vi "SPARK Create.vi"(8 "error in (no error)":errorcluster, 9 "Invert":bool, 10 "Device Number":u8) -> (0 "error out":errorcluster, 3 "MotorControlDeviceRef":T1={"DeviceStatus"={"status"=FALSE, "code"=0, "source"=""}, "Type"=enum."PWM", "PWM"={"PWM Channel"=enum."Invalid", "DeadBand"={"Name"="", "maxPositivePwm"=0, "minPositivePwm"=0, "centerPwm"=0, "maxNegativePwm"=0, "minNegativePwm"=0, "angularRange"=0}}, "CAN"={"Device Number"=0, "SetOutput VI Ref"=variant, "GetOutput VI Ref"=variant, "Enable VI Ref"=variant, "Disable VI Ref"=variant, "Data"=variant}, "Invert"=FALSE, "DIO PWM"={"PWM \"Enable\" Channel"=enum."Invalid", "DIOChannel"=enum."Invalid", "PWM Rate"=0.0}})   [LabVIEW 2023]
doc: "Open the SPARK motor controller.\n\n<b>Device Number</b> is the CAN ID of the controller. Use a value between 1 and 62.\n\n<b>Invert</b> will tell the LabVIEW driver to invert the output of the motor. For a device that is configured as a Follower, this flag will configure the follower to driver opposite of the Leader controller."
uses:
  <vilib>/Rock Robotics/WPI/MotorControl/WPI_MotorControlDeviceRef.ctl
  <vilib>/Rock Robotics/WPI/MotorControl/WPI_MotorControlType.ctl
  <vilib>/Rock Robotics/SystemInterfaces/DIO/FPGA_DIOPWMChannel.ctl
  <vilib>/Rock Robotics/WPI/PWM/WPI_PWMDeadband.ctl
  <vilib>/Rock Robotics/SystemInterfaces/DIO/FPGA_DIOChannel.ctl
  Typedef/Spark MAX Variant Data.ctl
  Typedef/SPARK Model.ctl
  Typedef/SPARK Parameter ID.ctl
  <vilib>/Rock Robotics/SystemInterfaces/NetworkCommunication/NetComm_UsageReport_ResourceType.ctl
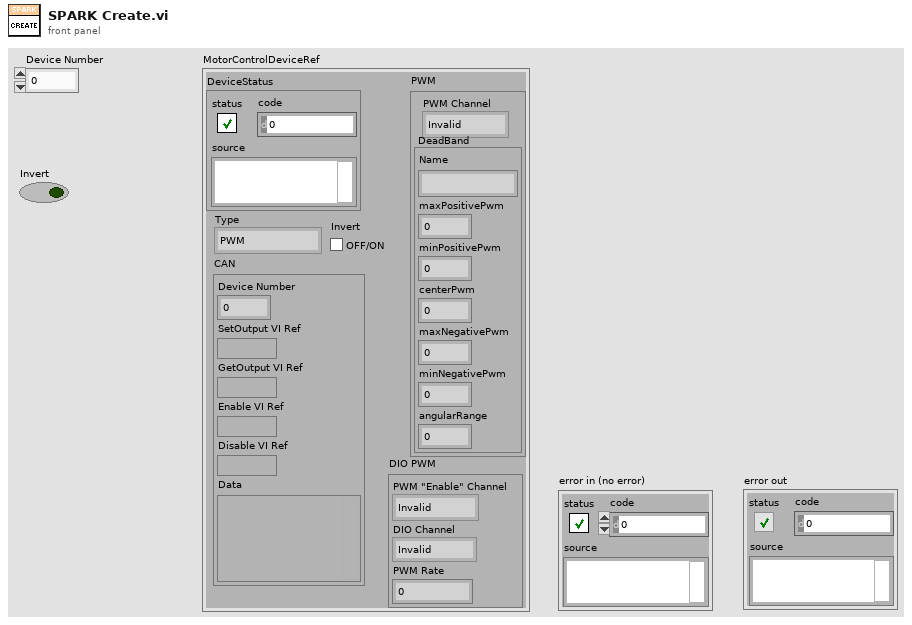
[diagram p1: front panel]
types:
  T1 = typedef "WPI_MotorControlDeviceRef.ctl" = cluster{"DeviceStatus":errorcluster, "Type":T2, "PWM":cluster{"PWM Channel":T3, "DeadBand":T4}, "CAN":cluster{"Device Number":u8, "SetOutput VI Ref":variant, "GetOutput VI Ref":variant, "Enable VI Ref":variant, "Disable VI Ref":variant, "Data":variant}, "Invert":bool, "DIO PWM":cluster{"PWM \"Enable\" Channel":T3, "DIOChannel":T5, "PWM Rate":dbl}}
  T2 = typedef "WPI_MotorControlType.ctl" = enum16{"PWM", "CAN", "DIO PWM"}
  T3 = typedef "FPGA_DIOPWMChannel.ctl" = enum8{"PWM 0", "PWM 1", "PWM 2", "PWM 3", "PWM 4", "PWM 5", "PWM 6", "PWM 7", "PWM 8", "PWM 9", "PWM MXP 0", "PWM MXP 1", "PWM MXP 2", "PWM MXP 3", "PWM MXP 4", "PWM MXP 5", "PWM MXP 6", "PWM MXP 7", "PWM MXP 8", "PWM MXP 9", "Invalid"}
  T4 = typedef "WPI_PWMDeadband.ctl" = cluster{"Name":string, "maxPositivePwm":i32, "minPositivePwm":i32, "centerPwm":i32, "maxNegativePwm":i32, "minNegativePwm":i32, "angularRange":u16}
  T5 = typedef "FPGA_DIOChannel.ctl" = enum8{"DIO 0", "DIO 1", "DIO 2", "DIO 3", "DIO 4", "DIO 5", "DIO 6", "DIO 7", "DIO 8", "DIO 9", "DIO MXP 0", "DIO MXP 1", "DIO MXP 2", "DIO MXP 3", "DIO MXP 4", "DIO MXP 5", "DIO MXP 6", "DIO MXP 7", "DIO MXP 8", "DIO MXP 9", "DIO MXP 10", "DIO MXP 11", "DIO MXP 12", "DIO MXP 13", "DIO MXP 14", "DIO MXP 15", "SPI Port CS1", "SPI Port CS2", "SPI Port CS3", "SPI Port MISO", "SPI Port MOSI", "Invalid"}
  T6 = typedef "SPARK Parameter ID.ctl" = enum16{"kCanID", "kInputMode", "kMotorType", "kCommAdvance", "kSensorType", "kCtrlType", "kIdleMode", "kInputDeadband", "kLegacyFeedbackSensorPID0", "kClosedLoopControlSensor", "kPolePairs", "kCurrentChop", "kCurrentChopCycles", "kP_0", "kI_0", "kD_0", "kF_0", "kIZone_0", "kDFilter_0", "kOutputMin_0", "kOutputMax_0", "kP_1", "kI_1", "kD_1", "kF_1", "kIZone_1", "kDFilter_1", "kOutputMin_1", "kOutputMax_1", "kP_2", "kI_2", "kD_2", "kF_2", "kIZone_2", "kDFilter_2", "kOutputMin_2", "kOutputMax_2", "kP_3", "kI_3", "kD_3", "kF_3", "kIZone_3", "kDFilter_3", "kOutputMin_3", "kOutputMax_3", "kInverted", "kOutputRatio", "kSerialNumberLow", "kSerialNumberMid", "kSerialNumberHigh", "kLimitSwitchFwdPolarity", "kLimitSwitchRevPolarity", "kHardLimitFwdEn", "kHardLimitRevEn", "kSoftLimitFwdEn", "kSoftLimitRevEn", "kRampRate", "kFollowerID", "kFollowerConfig", "kSmartCurrentStallLimit", "kSmartCurrentFreeLimit", "kSmartCurrentConfig", "kSmartCurrentReserved", "kMotorKv", "kMotorR", "kMotorL", "kMotorRsvd1", "kMotorRsvd2", "kMotorRsvd3", "kEncoderCountsPerRev", "kEncoderAverageDepth", "kEncoderSampleDelta", "kEncoderInverted", "kEncoderRsvd1", "kClosedLoopVoltageMode", "kCompensatedNominalVoltage", "kSmartMotionMaxVelocity_0", "kSmartMotionMaxAccel_0", "kSmartMotionMinVelOutput_0", "kSmartMotionAllowedClosedLoopError_0", "kSmartMotionAccelStrategy_0", "kSmartMotionMaxVelocity_1", "kSmartMotionMaxAccel_1", "kSmartMotionMinVelOutput_1", "kSmartMotionAllowedClosedLoopError_1", "kSmartMotionAccelStrategy_1", "kSmartMotionMaxVelocity_2", "kSmartMotionMaxAccel_2", "kSmartMotionMinVelOutput_2", "kSmartMotionAllowedClosedLoopError_2", "kSmartMotionAccelStrategy_2", "kSmartMotionMaxVelocity_3", "kSmartMotionMaxAccel_3", "kSmartMotionMinVelOutput_3", "kSmartMotionAllowedClosedLoopError_3", "kSmartMotionAccelStrategy_3", "kIMaxAccum_0", "kSlot3Placeholder1_0", "kSlot3Placeholder2_0", "kSlot3Placeholder3_0", "kIMaxAccum_1", "kSlot3Placeholder1_1", "kSlot3Placeholder2_1", "kSlot3Placeholder3_1", "kIMaxAccum_2", "kSlot3Placeholder1_2", "kSlot3Placeholder2_2", "kSlot3Placeholder3_2", "kIMaxAccum_3", "kSlot3Placeholder1_3", "kSlot3Placeholder2_3", "kSlot3Placeholder3_3", "kPositionConversionFactor", "kVelocityConversionFactor", "kClosedLoopRampRate", "kSoftLimitFwd", "kSoftLimitRev", "kSoftLimitRsvd0", "kSoftLimitRsvd1", "kAnalogPositionConversion", "kAnalogVelocityConversion", "kAnalogAverageDepth", "kAnalogSensorMode", "kAnalogInverted", "kAnalogSampleDelta", "kAnalogRsvd0", "kAnalogRsvd1", "kDataPortConfig", "kAltEncoderCountsPerRev", "kAltEncoderAverageDepth", "kAltEncoderSampleDelta", "kAltEncoderInverted", "kAltEncoderPositionConversion", "kAltEncoderVelocityConversion", "kAltEncoderRsvd0", "kAltEncoderRsvd1", "kHallSensorSampleRate", "kHallSensorAverageDepth", "kNumParameters", "kDutyCyclePositionFactor", "kDutyCycleVelocityFactor", "kDutyCycleInverted", "kDutyCycleSensorMode", "kDutyCycleAverageDepth", "kDutyCycleSampleDelta", "kDutyCycleOffsetv1p6p2", "kDutyCycleRsvd0", "kDutyCycleRsvd1", "kDutyCycleRsvd2", "kPositionPIDWrapEnable", "kPositionPIDMinInput", "kPositionPIDMaxInput", "kDutyCycleZeroCentered", "kDutyCyclePrescalar", "kDutyCycleOffset", "kProductId", "kDeviceMajorVersion", "kDeviceMinorVersion", "kStatus0Period", "kStatus1Period", "kStatus2Period", "kStatus3Period", "kStatus4Period", "kStatus5Period", "kStatus6Period", "kStatus7Period", "kMAXMotionMaxVelocity_0", "kMAXMotionMaxAccel_0", "kMAXMotionMaxJerk_0", "kMAXMotionAllowedClosedLoopError_0", "kMAXMotionPositionMode_0", "kMAXMotionMaxVelocity_1", "kMAXMotionMaxAccel_1", "kMAXMotionMaxJerk_1", "kMAXMotionAllowedClosedLoopError_1", "kMAXMotionPositionMode_1", "kMAXMotionMaxVelocity_2", "kMAXMotionMaxAccel_2", "kMAXMotionMaxJerk_2", "kMAXMotionAllowedClosedLoopError_2", "kMAXMotionPositionMode_2", "kMAXMotionMaxVelocity_3", "kMAXMotionMaxAccel_3", "kMAXMotionMaxJerk_3", "kMAXMotionAllowedClosedLoopError_3", "kMAXMotionPositionMode_3", "kForceEnableStatus0", "kForceEnableStatus1", "kForceEnableStatus2", "kForceEnableStatus3", "kForceEnableStatus4", "kForceEnableStatus5", "kForceEnableStatus6", "kForceEnableStatus7", "kFollowerModeLeaderId", "kFollowerModeIsInverted", "kDutyCycleEncoderStartPulseUs", "kDutyCycleEncoderEndPulseUs"}
  T7 = typedef "Spark MAX Variant Data.ctl" = cluster{"Ext ID":u32, "CAN Timeout":u32, "Inverted No WPILib":bool, "Has Configured Limit Sw":bool, "Has Configured Alt Encoder":bool, "SPARK Model":T8, "CAN Max Retries":u32, "CAN Timeout (ms)":u32, "Status 0 Period (ms)":u32, "Status 1 Period (ms)":u32, "Status 2 Period (ms)":u32, "Status 3 Period (ms)":u32, "Status 4 Period (ms)":u32, "Status 5 Period (ms)":u32, "Status 6 Period (ms)":u32, "Status 7 Period (ms)":u32, "Status Frame Timeout (ms)":u32}
  T8 = typedef "SPARK Model.ctl" = enum16{"SPARK MAX", "SPARK Flex", "Unknown"}
  T9 = cluster{"Device Number":u8, "SetOutput VI Ref":variant, "GetOutput VI Ref":variant, "Enable VI Ref":variant, "Disable VI Ref":variant, "Data":variant}
  T10 = typedef "SPARK Firmware Version.ctl" = cluster{"Major":u8, "Minor":u8, "Build":u16, "Version String":string}
  T11 = typedef "NetComm_UsageReport_ResourceType.ctl" = enum8{"Controller", "Module", "Language", "CANPlugin", "Accelerometer", "ADXL345", "AnalogChannel", "AnalogTrigger", "AnalogTriggerOutput", "CANJaguar", "Compressor", "Counter", "Dashboard", "DigitalInput", "DigitalOutput", "DriverStationCIO", "DriverStationEIO", "DriverStationLCD", "Encoder", "GearTooth", "Gyro", "I2C", "Framework", "Jaguar", "Joystick", "Kinect", "KinectStick", "PIDController", "Preferences", "PWM", "Relay", "RobotDrive", "SerialPort", "Servo", "Solenoid", "SPI", "Task", "Ultrasonic", "Victor", "Button", "Command", "AxisCamera", "PCVideoServer", "SmartDashboard", "Talon", "HiTechnicColorSensor", "HiTechnicAccel", "HiTechnicCompass", "SRF08", "AnalogOutput", "Victor SP", "Talon SRX", "CAN Talon SRX", "ADXL362 Accel", "ADXRS450 Gyro", "Rev SPARK", "Mindsensors SD540", "Digital Filter", "ADIS16448", "PDP", "PCM", "PigeonIMU", "Nidec Brushless", "CTRE CANifier", "CTRE TalonFX", "CTRE Future 1", "CTRE Future 2", "CTRE Future 3", "CTRE Future 4", "CTRE Future 5", "CTRE Future 6", "Linear Filter", "Xbox Controller", "USB Camera", "NavX", "Pixy", "Pixy2", "ScanseSweep", "Shuffleboard", "CAN", "Digilent DMC60", "PWM Victor SPX", "Rev SPARK MAX PWM", "Rev SPARK MAX CAN", "ADIS16470", "PIDController2", "ProfiledPIDController", "Kinematics", "Odometry", "Units", "Trapezoid Profile", "DutyCycle", "Addressable LEDs", "Fusion Venom", "CTRE Future 7", "CTRE Future 8", "CTRE Future 9", "CTRE Future 10", "CTRE Future 11", "CTRE Future 12", "CTRE Future 13", "CTRE Future 14", "Exponential Profile", "PS4 Controller", "Photon Camera", "Photon Pose Estimator", "Path Planner Path", "Path Planner Auto", "Path Finding Command", "Redux Future 1", "Redux Future 2", "Redux Future 3", "Redux Future 4", "Redux Future 5", "Rev SPARK Flex CAN", "Rev SPARK Flex PWM"}
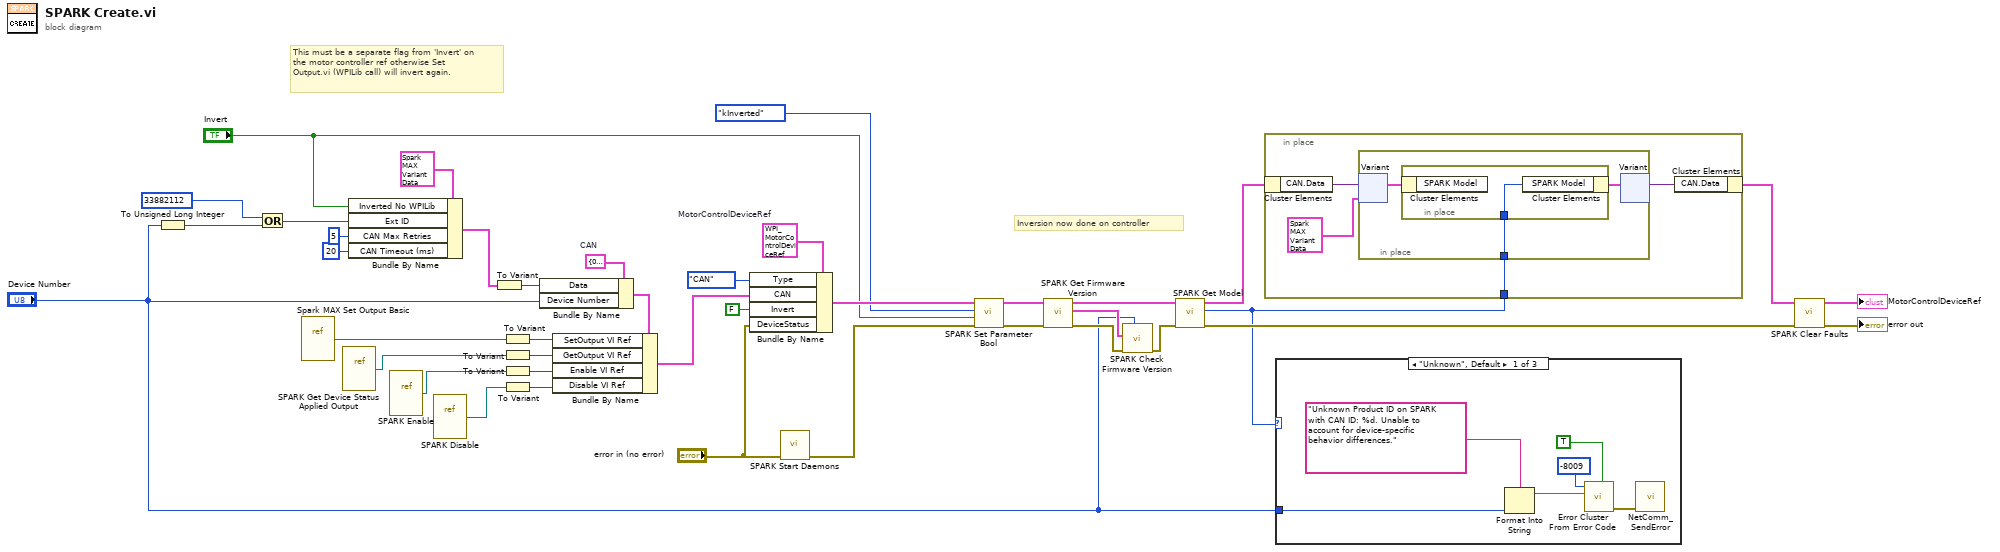
[diagram p0: block diagram]
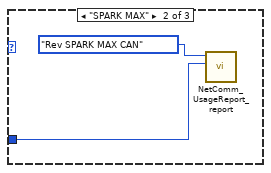
[diagram p2: hidden frame]
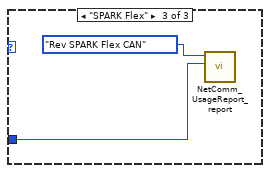
[diagram p3: hidden frame]
diagram:
  w35 = T9 {"Device Number"=0, "SetOutput VI Ref"=variant, "GetOutput VI Ref"=variant, "Enable VI Ref"=variant, "Disable VI Ref"=variant, "Data"=variant}  # CAN
  w33 = T1 {"DeviceStatus"={"status"=FALSE, "code"=0, "source"=""}, "Type"=enum."PWM", "PWM"={"PWM Channel"=enum."Invalid", "DeadBand"={"Name"="", "maxPositivePwm"=0, "minPositivePwm"=0, "centerPwm"=0, "maxNegativePwm"=0, "minNegativePwm"=0, "angularRange"=0}}, "CAN"={"Device Number"=0, "SetOutput VI Ref"=variant(refnum<vi> refnum), "GetOutput VI Ref"=variant(refnum<vi> refnum), "Enable VI Ref"=variant(refnum<vi> refnum), "Disable VI Ref"=variant(refnum<vi> refnum), "Data"=variant}, "Invert"=FALSE, "DIO PWM"={"PWM \"Enable\" Channel"=enum."Invalid", "DIOChannel"=enum."Invalid", "PWM Rate"=0.0}}  # MotorControlDeviceRef
  # "This must be a separate flag from 'Invert' on the motor controller ref otherwise Set Output.vi (WPILib call) will invert again."
  # "Inversion now done on controller"
  n1 = To Unsigned Long Integer(number="Device Number") -> (unsigned 32bit integer=w38:u32)
  n2 = Or(x=u32 33882112 ("MotorCtrl | REV"), y=w38) -> (x .or. y?=w23:u32)
  n3 = vi-ref "Spark MAX Set Output Basic.vi"() -> (w31:refnum<vi>)
  n4 = vi-ref "SPARK Get Device Status Applied Output.vi"() -> (w29:refnum<vi>)
  n5 = Bundle By Name(cluster=T7 {"Ext ID"=0, "CAN Timeout"=0, "Inverted No WPILib"=FALSE, "Has Configured Limit Sw"=FALSE, "Has Configured Alt Encoder"=FALSE, "SPARK Model"=enum."Unknown", "CAN Max Retries"=5, "CAN Timeout (ms)"=20, "Status 0 Period (ms)"=10, "Status 1 Period (ms)"=250, "Status 2 Period (ms)"=20, "Status 3 Period (ms)"=20, "Status 4 Period (ms)"=20, "Status 5 Period (ms)"=20, "Status 6 Period (ms)"=20, "Status 7 Period (ms)"=20, "Status Frame Timeout (ms)"=500}, "Inverted No WPILib"="Invert", "Ext ID"=w23, "CAN Max Retries"=u32 5, "CAN Timeout (ms)"=u32 20) -> (w39:T7)
  n6 = vi-ref "SPARK Enable.vi"() -> (w27:refnum<vi>)
  n7 = vi-ref "SPARK Disable.vi"() -> (w26:refnum<vi>)
  n8 = To Variant(anything=w39) -> (Variant=w40:variant)
  n9 = To Variant(anything=w31) -> (Variant=w30:variant)
  n10 = To Variant(anything=w29) -> (Variant=w28:variant)
  n11 = To Variant(anything=w27) -> (Variant=w25:variant)
  n12 = To Variant(anything=w26) -> (Variant=w24:variant)
  n13 = Bundle By Name(cluster=w35, "Data"=w40, "Device Number"="Device Number") -> (w36:T9)
  n14 = Bundle By Name(cluster=w36, "SetOutput VI Ref"=w30, "GetOutput VI Ref"=w28, "Enable VI Ref"=w25, "Disable VI Ref"=w24) -> (w32:T9)
  n15 = Bundle By Name(cluster=w33, "Type"=WPI_MotorControlType."CAN", "CAN"=w32, "Invert"=FALSE, "DeviceStatus"="error in (no error)") -> (w22:T1)
  n16 = call "SPARK Start Daemons.vi"("error in (no error)"="error in (no error)") -> ("error out"=w9:errorcluster)  [unwired: 10 in]
  n17 = call "SPARK Set Parameter Bool.vi"("error in (no error)"=w9, "Boolean (F)"="Invert", "Parameter ID"=SPARK_Parameter_ID."kInverted", "MotorControlDeviceRef"=w22) -> ("error out"=w10:errorcluster, "MotorControlDeviceRef"=w11:T1)  [unwired: 6 in]
  n18 = call "SPARK Get Firmware Version.vi"("error in (no error)"=w10, "MotorControlDeviceRef in"=w11) -> ("error out"=w14:errorcluster, "Firmware Version"=w15:T10, "MotorControlDeviceRef out"=w12:T1)  [unwired: 5 in, 2 out]
  n19 = call "SPARK Check Firmware Version.vi"("CAN ID"="Device Number", "error in (no error)"=w14, "Firmware Version"=w15) -> ("error out"=w13:errorcluster)  [unwired: 8 in]
  n20 = call "SPARK Get Model.vi"("error in (no error)"=w13, "MotorControlDeviceRef in"=w12) -> ("error out"=w16:errorcluster, "SPARK Model"=w4:T8, "MotorControlDeviceRef"=w5:T1)  [unwired: 7 in]
  n21 = in-place {
    in-place-border: w4 -> [w42]
    n22 = in-place-cluster #1(w5) -> ("CAN.Data"=w43:variant)
    n23 = in-place {
      in-place-border: w42 -> [w46]
      n24 = in-place-variant #2(w43, T7 {"Ext ID"=0, "CAN Timeout"=0, "Inverted No WPILib"=FALSE, "Has Configured Limit Sw"=FALSE, "Has Configured Alt Encoder"=FALSE, "SPARK Model"=enum."Unknown", "CAN Max Retries"=5, "CAN Timeout (ms)"=20, "Status 0 Period (ms)"=10, "Status 1 Period (ms)"=250, "Status 2 Period (ms)"=20, "Status 3 Period (ms)"=20, "Status 4 Period (ms)"=20, "Status 5 Period (ms)"=20, "Status 6 Period (ms)"=20, "Status 7 Period (ms)"=20, "Status Frame Timeout (ms)"=500}) -> (w47:T7)  [unwired: 1 out]
      n25 = in-place {
        in-place-border: w46 -> [w48]
        n26 = in-place-cluster #3(w47) -> ()  [unwired: 1 out]
        n27 = in-place-cluster #3("SPARK Model"=w48) -> (w45:T7)
      }
      n28 = in-place-variant #2(w45) -> (w41:variant)  [unwired: 1 out]
    }
    n29 = in-place-cluster #1("CAN.Data"=w41) -> (w3:T1)
  }
  n30 = case shown="\"Unknown\", Default" w4 {
    tunnel: "Device Number" -> [w49 w55 w57]
    frame "Unknown", Default {
      n31 = Format Into String(format string="Unknown Product ID on SPARK with CAN ID: %d. Unable to account for device-specific behavior differences.", w49) -> (resulting string=w54:string)  [unwired: 2 in, 1 out]
      n32 = call <vilib>:"Error Cluster From Error Code.vi"("is warning? (False)"=TRUE, "error message (\"\")"=w54, "error code (0)"=-8009) -> ("error out"=w50:errorcluster)  [unwired: 6 in]
      n33 = call <vilib>:"NetComm_SendError.vi"("error in (no error)"=w50) -> ()  [unwired: 11 in]
    }
    frame "SPARK MAX" {
      n34 = call <vilib>:"NetComm_UsageReport_report.vi"("Instance Number"=w55, "Resource Type"=NetComm_UsageReport_ResourceType."Rev SPARK MAX CAN") -> ()  [unwired: 10 in]
    }
    frame "SPARK Flex" {
      n35 = call <vilib>:"NetComm_UsageReport_report.vi"("Instance Number"=w57, "Resource Type"=NetComm_UsageReport_ResourceType."Rev SPARK Flex CAN") -> ()  [unwired: 10 in]
    }
  }
  n36 = call "SPARK Clear Faults.vi"("error in"=w16, "MotorControlDeviceRef"=w3) -> ("error out"=→"error out":errorcluster, "MotorControlDeviceRef"=→"MotorControlDeviceRef":T1)  [unwired: 8 in]
